vi "Ramp_SubVI.vi"(0 "Enum":enum16{"linear", "power"}(ring), 3 "index":i32, 4 "step":dbl, 5 "end":dbl, 6 "start":dbl) -> (1 "Stop?":bool, 2 "Numeric":dbl)   [LabVIEW 2010]
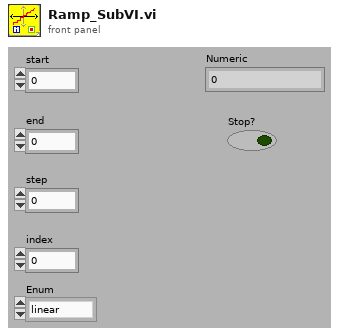
[diagram p1: front panel]
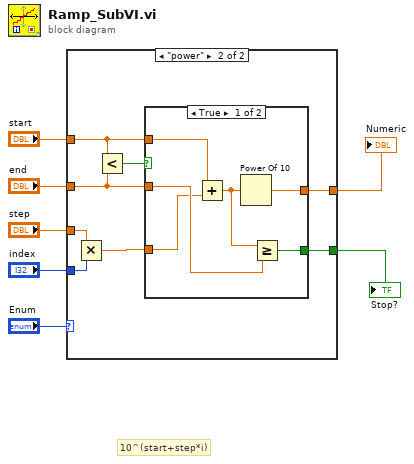
[diagram p0: block diagram]
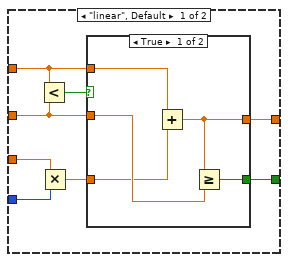
[diagram p2: hidden frame]
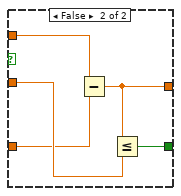
[diagram p3: hidden frame]
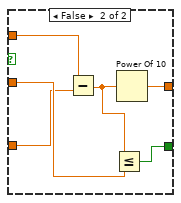
[diagram p4: hidden frame]
diagram:
  # "10^(start+step*i)"
  n1 = case shown="\"power\"" "Enum" {
    tunnel: "end" -> [w15 w33]
    tunnel: "start" -> [w14 w32]
    tunnel: [w13 w31] -> w5
    tunnel: "step" -> [w10 w28]
    tunnel: "index" -> [w9 w27]
    tunnel: [w11 w29] -> w2
    frame "linear", Default {
      n2 = Less?(x=w14, y=w15) -> (x < y?=w12:bool)
      n3 = Multiply(x=w10, y=w9) -> (x*y=w8:dbl)
      n4 = case shown="True" w12 {
        tunnel: w14 -> [w20 w25]
        tunnel: [w19 w24] -> w11
        tunnel: w15 -> [w18 w23]
        tunnel: [w17 w22] -> w13
        tunnel: w8 -> [w16 w21]
        frame True {
          n5 = Add(x=w20, y=w16) -> (x+y=w19:dbl)
          n6 = Greater Or Equal?(x=w19, y=w18) -> (x >= y?=w17:bool)
        }
        frame False {
          n7 = Subtract(x=w25, y=w21) -> (x-y=w24:dbl)
          n8 = Less Or Equal?(x=w24, y=w23) -> (x <= y?=w22:bool)
        }
      }
    }
    frame "power" {
      n9 = Multiply(x=w28, y=w27) -> (x*y=w26:dbl)
      n10 = Less?(x=w32, y=w33) -> (x < y?=w30:bool)
      n11 = case shown="True" w30 {
        tunnel: w32 -> [w39 w45]
        tunnel: [w35 w41] -> w29
        tunnel: w33 -> [w38 w44]
        tunnel: [w37 w43] -> w31
        tunnel: w26 -> [w36 w42]
        frame True {
          n12 = Add(x=w39, y=w36) -> (x+y=w34:dbl)
          n13 = Power Of 10(x=w34) -> (10^x=w35:dbl)
          n14 = Greater Or Equal?(x=w34, y=w38) -> (x >= y?=w37:bool)
        }
        frame False {
          n15 = Subtract(x=w45, y=w42) -> (x-y=w40:dbl)
          n16 = Less Or Equal?(x=w40, y=w44) -> (x <= y?=w43:bool)
          n17 = Power Of 10(x=w40) -> (10^x=w41:dbl)
        }
      }
    }
  }
  "Numeric" <- w2
  "Stop?" <- w5
